vi "array_to_string.vi"(1 "Void_param":dbl[](array[numeric])) -> (0 "String":string)   [LabVIEW 2016]
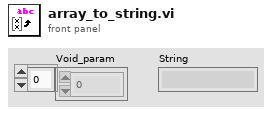
[diagram p1: front panel]
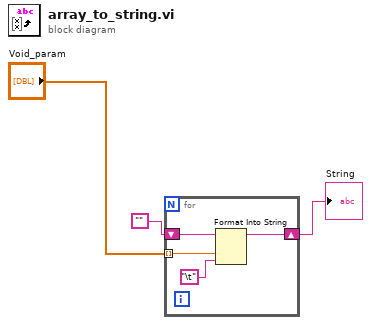
[diagram p0: block diagram]
diagram:
  n1 = for {
    tunnel: "Void_param" -> [w7] mode=indexing
    shift-right: [w6] -> w2
    shift-left: "" -> [w4]
    n2 = Format Into String(initial string=w4, w7, "\t") -> (resulting string=w6:string)  [unwired: 2 in, 1 out]
  }
  "String" <- w2
